vi "Element Init.vi"(7 "VolatusAPI":refnum<class "VolatusAPI.lvclass">, 8 "error in (no error)":errorcluster, 10 "JSON":string, 11 "DoubleControl in":refnum<class "SliderControl.lvclass">) -> (0 "error out":errorcluster, 3 "DoubleControl out":refnum<class "SliderControl.lvclass">)   [LabVIEW 2020, in "VolatusGUIElements.lvlib" / "SliderControl.lvclass"]
uses:
  SliderControl.lvclass
  C:/dev/lv20CE/relink/lv-volatus/VolatusGUI/GUI Element/GUI Element.lvclass
  Volatus/VolatusAPI/VolatusAPI.lvclass
  JSON.ctl
  VolatusGUI/GUI Element/GUI Element.lvclass/GUI Element.ctl
  lv-vecto/Vecto/Group DBL/Group DBL.lvclass
  C:/dev/lv20CE/relink/lv-vecto/Vecto/Group/Group.lvclass
  SliderControl.lvclass/SliderControl.ctl
  9f5f9d7c-72d9-4199-bc14-3b816086c6b7.vi
  <vilib>/JDP Science/JSONtext/JSON text to Variant.vi
  <vilib>/JDP Science/JSONtext/LVClass Serializer/JSONtext LVClass Serializer.lvclass
  lv-vecto/Vecto/Channel DBL/Channel DBL.lvclass
  VolatusGUI/GUI Element/GUI Element.lvclass
  VolatusGUI/Element Inhibit/Element Inhibit.lvclass
  Volatus/Numeric Command/Numeric Command.lvclass
  C:/dev/lv20CE/relink/lv-vecto/Vecto/Group DBL/Group DBL.lvclass
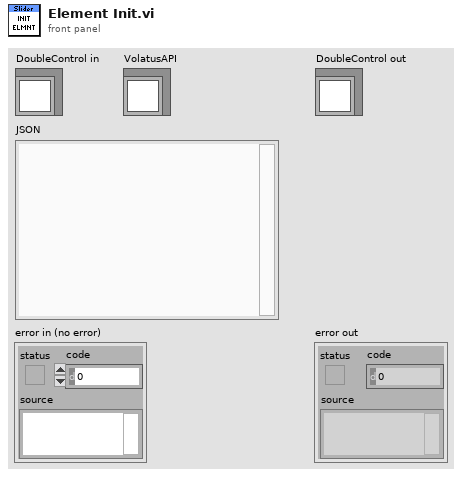
[diagram p1: front panel]
types:
  T1 = typedef "VolatusGUIElements.lvlib/SliderControl.lvclass/JSON.ctl" = cluster{"Channel":string, "Staleness":dbl, "Inhibit":string}
  T2 = typedef "VectoConfig.lvlib/Channel Info.ctl" = cluster{"Name":string, "Group":string, "Owning Node":string, "Owning Task":string, "Resource":string}
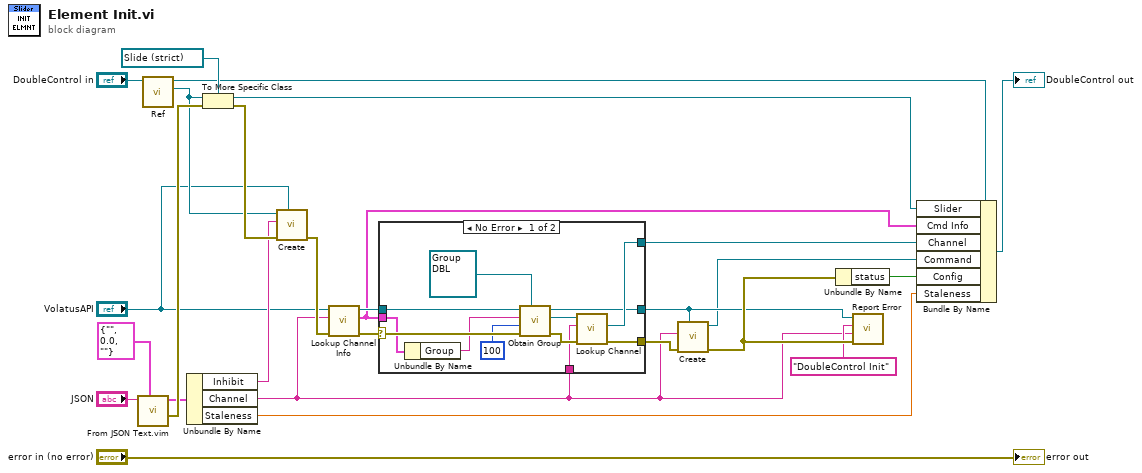
[diagram p0: block diagram]
diagram:
  n1 = call "From JSON Text.vim"("Data Type and Default Value"=T1 {"Channel"="", "Staleness"=0.0, "Inhibit"=""} ("JSON"), "JSON"="JSON") -> ("error out"=w24:errorcluster, "Data out"=w17:T1)  [unwired: 8 in]
  n2 = call "Ref.vi"("GUI Element in"="DoubleControl in") -> ("Ref"=w5:refnum<vi>, "GUI Element out"=w10:refnum<class "SliderControl.lvclass">)  [unwired: 9 in]
  n3 = Unbundle By Name(w17) -> ("Inhibit"=w6:string, "Channel"=w3:string, "Staleness"=w8:dbl)
  n4 = To More Specific Class(target class=refnum<vi> refnum ("Vertical Pointer Slide"), reference=w5, error in=w24) -> (specific class reference=w9:refnum<vi>, error out=w25:errorcluster)
  n5 = call "Create.vi"("VolatusAPI"="VolatusAPI", "error in (no error)"=w25, "Inhibit Channel"=w6, "Control Ref"=w5) -> ("error out"=w23:errorcluster)  [unwired: 6 in, 1 out]
  n6 = call "Lookup Channel Info.vi"("error in (no error)"=w23, "Channel Name"=w3, "VolatusAPI in"="VolatusAPI") -> ("error out"=w22:errorcluster, "Channel Info"=w7:T2, "VolatusAPI out"=w16:refnum<class "VolatusAPI.lvclass">)  [unwired: 5 in, 1 out]
  n7 = case shown="No Error" w22 {
    selector: w22 -> [w38 w40]
    tunnel: [w39 w40] -> w26
    tunnel: w16 -> [w36 w41]
    tunnel: [w32 _] -> w14
    tunnel: [w31 w41] -> w2
    tunnel: w3 -> [w30 _]
    tunnel: w7 -> [w29 _]
    frame No Error {
      n8 = Unbundle By Name(w29) -> ("Group"=w37:string)
      n9 = call "Obtain Group.vi"("Group Type (Abstract)"=refnum<class "Group DBL.lvclass"> refnum ("Vecto.lvlib:Group.lvclass"), "error in (no error)"=w38, "Timeout ms (5000)"=u32 100, "Group Name"=w37, "VolatusAPI in"=w36) -> ("error out"=w33:errorcluster, "Group"=w34:refnum<class "Group DBL.lvclass">, "VolatusAPI out"=w31:refnum<class "VolatusAPI.lvclass">)  [unwired: 4 in]
      n10 = call "Lookup Channel.vi"("error in (no error)"=w33, "Channel Name"=w30, "Group in"=w34) -> ("error out"=w39:errorcluster, "Channel"=w32:refnum<class "Channel DBL.lvclass">)  [unwired: 6 in, 1 out]
    }
    frame Error {
    }
  }
  n11 = call "Create.vi"("VolatusAPI"=w2, "error in (no error)"=w26, "Channel"=w3) -> ("error out"=w27:errorcluster, "Numeric Command out"=w1:refnum<class "Numeric Command.lvclass">)  [unwired: 7 in]
  n12 = Unbundle By Name(w27) -> ("status"=w13:bool)
  n13 = call "Report Error.vi"("error in (no error)"=w27, "Message"=w3, "Context"="DoubleControl Init", "VolatusAPI in"=w2) -> ()  [unwired: 6 in, 2 out]
  n14 = Bundle By Name(cluster=w10, "Slider"=w9, "Cmd Info"=w7, "Channel"=w14, "Command"=w1, "Config"=w13, "Staleness"=w8) -> (→"DoubleControl out":refnum<class "SliderControl.lvclass">)
  "error out" <- "error in (no error)"
